vi "DER_VF_subTest.vi"(7 "Test Result in":T2=enum."Success", 8 "error in":errorcluster, 9 "DeviceID":T1, 10 "MicrogridID":u8, 11 "Message Enqueuer in":refnum<class "Message Enqueuer.lvclass">) -> (0 "error out":errorcluster, 1 "dup DeviceID":T1, 2 "dup MicrogridID":u8, 3 "Message Enqueuer out":refnum<class "Message Enqueuer.lvclass">, 5 "Test Result out":T2=enum."Success")   [LabVIEW 2018, in "IED Test Framework.lvlib" / "IED Test.lvclass"]
uses:
  IED Test.lvclass
  <vilib>/ActorFramework/Message Enqueuer/Message Enqueuer.lvclass
  Controls/Test Result.ctl
  <vilib>/ORNL/CSEISMIC DDS/CSEISMIC DDS Base/Data Types/Controls/DeviceID.ctl
  <vilib>/ORNL/CSEISMIC DDS/CSEISMIC DDS Base/Data Types/DER_VF.ctl
  <vilib>/ORNL/CSEISMIC DDS/CSEISMIC DDS Base/CSEISMIC DDS.lvclass/CSEISMIC DDS.ctl
  DER Actor/DER Messages/Write DER VF Msg/Write DER VF Msg.lvclass/Write DER VF Msg.ctl
  <vilib>/ActorFramework/Message Enqueuer/Message Enqueuer.lvclass/Message Enqueuer.ctl
  <vilib>/ORNL/CSEISMIC DDS/CSEISMIC DDS Base/Accessors/Write DDS Reference.vi
  <vilib>/ActorFramework/Message Enqueuer/Enqueue.vi
  <vilib>/ORNL/CSEISMIC DDS/CSEISMIC DDS Base/Accessors/Read DDS Reference.vi
  <vilib>/ORNL/CSEISMIC DDS/DDS Reader/DDS Reader.lvclass
  C:/Program Files (x86)/National Instruments/LabVIEW 2018/vi.lib/ORNL/CSEISMIC DDS/CSEISMIC DDS Base/CSEISMIC DDS.lvclass
  DER Actor/DER Messages/Write DER VF Msg/Write DER VF Msg.lvclass
  C:/Program Files (x86)/National Instruments/LabVIEW 2018/vi.lib/ActorFramework/Message/Message.lvclass
  <vilib>/ORNL/CSEISMIC DDS/CSEISMIC DDS Base/Error Handler.vi
  <vilib>/ActorFramework/Message Priority Queue/Priority Enqueue.vi
  <vilib>/ORNL/CSEISMIC DDS/CSEISMIC DDS Base/CSEISMIC DDS.lvclass
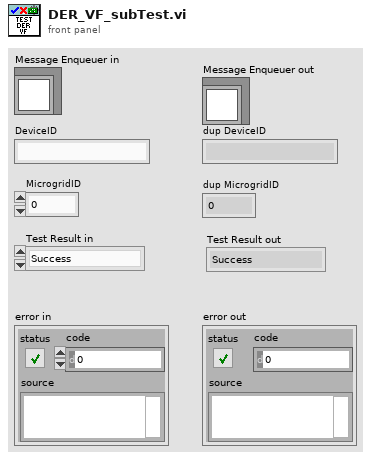
[diagram p1: front panel]
types:
  T1 = typedef "CSEISMIC DDS.lvlib/CSEISMIC DDS.lvclass/DeviceID.ctl" = string
  T2 = typedef "IED Test Framework.lvlib/IED Test.lvclass/Test Result.ctl" = enum16{"Invalid", "Success", "Failure", "Error", "Timeout"}
  T3 = typedef "CSEISMIC DDS.lvlib/CSEISMIC DDS.lvclass/DER_VF.ctl" = cluster{"DeviceID":T1}
  T4 = typedef "LVDDS_library.lvlib/DDS Sample Info.ctl" = cluster{"DDS_SampleStateKind":enum32{"DDS_INVALID_SAMPLE_STATE", "DDS_READ_SAMPLE_STATE", "DDS_NOT_READ_SAMPLE_STATE"}, "DDS_ViewStateKind":enum32{"DDS_INVALID_SAMPLE_STATE", "DDS_NEW_VIEW_STATE", "DDS_NOT_NEW_VIEW_STATE"}, "DDS_InstanceStateKind":enum32{"DDS_INVALID_STATE", "DDS_ALIVE_INSTANCE_STATE", "DDS_NOT_ALIVE_DISPOSED_INSTANCE_STATE", "", "DDS_NOT_ALIVE_NO_WRITERS_INSTANCE_STATE"}, "sec":i32, "nanosec":u32, "valid_data":bool}
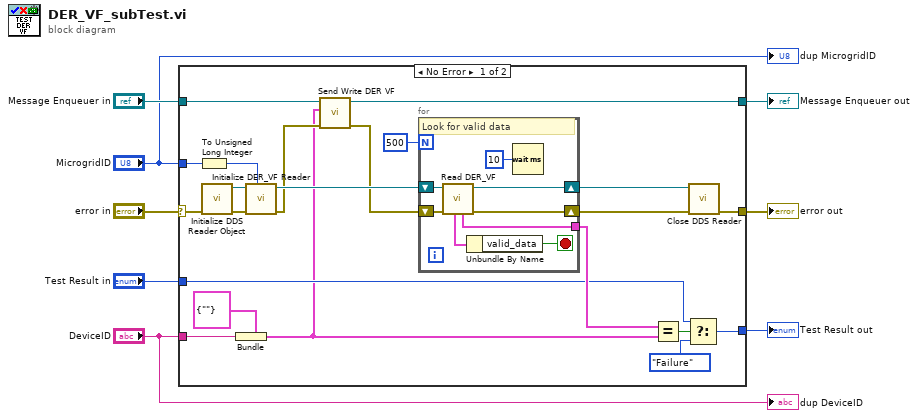
[diagram p0: block diagram]
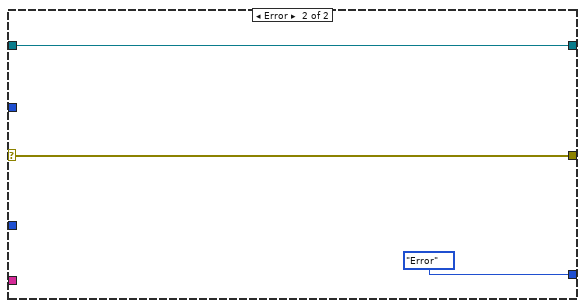
[diagram p2: hidden frame]
diagram:
  n1 = case shown="No Error" "error in" {
    selector: "error in" -> [w25 w40]
    tunnel: [w30 Test_Result."Error" ("Test Result")] -> w2
    tunnel: "DeviceID" -> [w10 _]
    tunnel: [w12 w39] -> w4
    tunnel: [w20 w40] -> w3
    tunnel: "Message Enqueuer in" -> [w13 w39]
    tunnel: "Test Result in" -> [w26 _]
    tunnel: "MicrogridID" -> [w16 _]
    frame No Error {
      n2 = To Unsigned Long Integer(number=w16) -> (unsigned 32bit integer=w19:u32)
      n3 = call <vilib>:"Initialize DDS Reader Object.vi"("error in"=w25) -> ("error out"=w24:errorcluster, "DDS Reader out"=w23:refnum<class "DDS Reader.lvclass">)  [unwired: 9 in]
      n4 = Bundle(cluster=T3 {"DeviceID"=""} ("DER_VF"), "DeviceID"=w10) -> (w9:T3)
      n5 = call <vilib>:"Initialize DER_VF Reader.vi"("MicrogridID"=w19, "error in"=w24, "DDS Reader in"=w23) -> ("error out"=w15:errorcluster, "DDS Reader out"=w21:refnum<class "DDS Reader.lvclass">)  [unwired: 7 in]
      n6 = call "Send Write DER VF.vi"("error in (no error)"=w15, "DER_VF"=w9, "Message Enqueuer"=w13) -> ("error out"=w14:errorcluster, "Message Enqueuer out"=w12:refnum<class "Message Enqueuer.lvclass">)  [unwired: 7 in]
      n7 = for {
        N: 500 -> [_]
        tunnel: [w35] -> w27
        shift-right: [w37] -> w22
        shift-left: w14 -> [w38]
        shift-right: [w34] -> w17
        shift-left: w21 -> [w36]
        stop <- w31 stop-if-true
        # "Look for valid data"
        n8 = call <vilib>:"Read DER_VF.vi"("error in"=w38, "DDS Reader in"=w36) -> ("error out"=w37:errorcluster, "DDS Reader out"=w34:refnum<class "DDS Reader.lvclass">, "data"=w35:T3, "DDS Sample Info"=w32:T4)  [unwired: 6 in]
        n9 = Unbundle By Name(w32) -> ("valid_data"=w31:bool)
        n10 = Wait (ms)(milliseconds to wait=u32 10) -> ()  [unwired: 1 out]
      }
      n11 = Equal?(x=w27, y=w9) -> (x = y?=w28:bool)
      n12 = Select(t=w26, s=w28, f=Test_Result."Failure" ("Test Result")) -> (s? t:f=w30:T2)
      n13 = call <vilib>:"Close DDS Reader.vi"("error in"=w22, "DDS Reader in"=w17) -> ("error out"=w20:errorcluster)  [unwired: 9 in]
    }
    frame Error {
    }
  }
  "Test Result out" <- w2
  "error out" <- w3
  "Message Enqueuer out" <- w4
  "dup DeviceID" <- "DeviceID"
  "dup MicrogridID" <- "MicrogridID"
